vi "Get VIDoc Settings Path.vi"(8 "error in (no error)":errorcluster {"code" format="Error %.0f"}, 11 "VIDoc Settings In":refnum<class "VIDoc Settings.lvclass">) -> (0 "error out":errorcluster {"code" format="Error %.0f"}, 2 "VIDoc Settings Path":path, 3 "VIDoc Settings Out":refnum<class "VIDoc Settings.lvclass">)   [LabVIEW 2023, in "VIDoc Settings.lvclass"]
uses:
  VIDoc Settings.lvclass
  VIDoc Settings.lvclass/VIDoc Settings.ctl
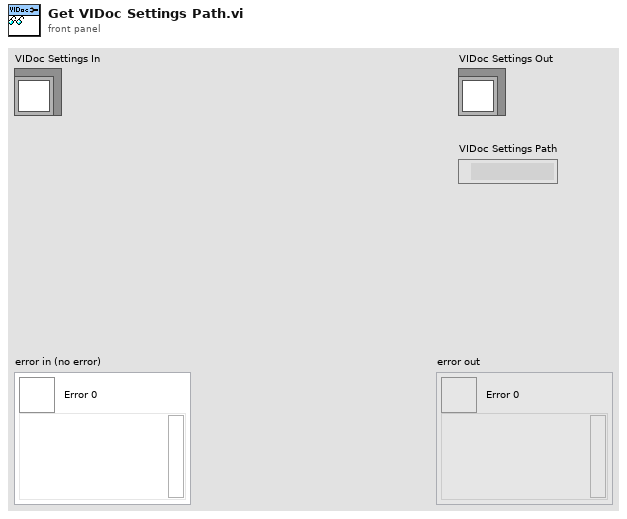
[diagram p1: front panel]
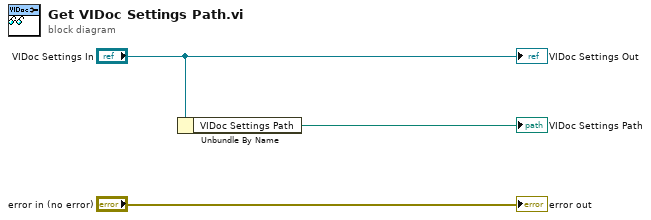
[diagram p0: block diagram]
diagram:
  n1 = Unbundle By Name("VIDoc Settings In") -> ("VIDoc Settings Path"=→"VIDoc Settings Path":path)
  "error out" <- "error in (no error)"
  "VIDoc Settings Out" <- "VIDoc Settings In"
